vi "TDT-Stream AO.vi"(0 "RPcox":refnum<k7>, 2 "Action":T1=enum."Write", 5 "Restart":bool, 7 "Output array":dbl[][](array[numeric]), 9 "Chans":i32[](array[numeric]), 11 "error in (no error)":errorcluster) -> (4 "RPcox thru":refnum<k7>, 15 "error out":errorcluster={"status"=FALSE, "code"=0, "source"="."})   [LabVIEW 2020]
uses:
  TDT-Signal Bank Action.ctl
  TDT-Globals.vi
  Utility VIs/Array Manipulation VIs/Array-Dimensions (2D).vi
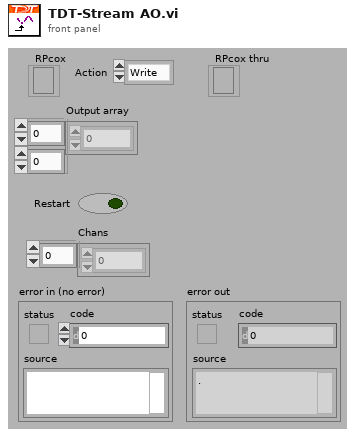
[diagram p1: front panel]
types:
  T1 = typedef "TDT-Signal Bank Action.ctl" = enum16{"Init", "Write", "Read", "Rewrite", "Reset", "Recycle", "Ramp up", "Ramp down", "Zero"}
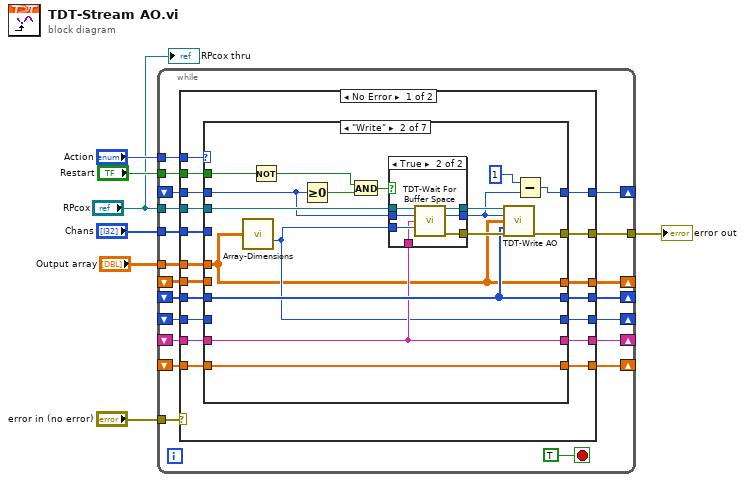
[diagram p0: block diagram]
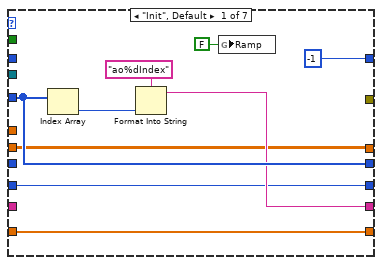
[diagram p2: hidden frame]
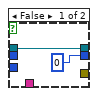
[diagram p3: hidden frame]
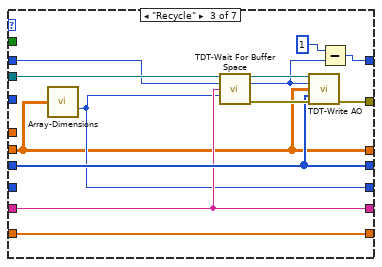
[diagram p4: hidden frame]
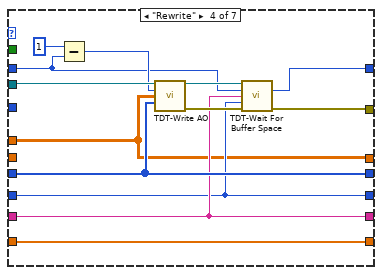
[diagram p5: hidden frame]
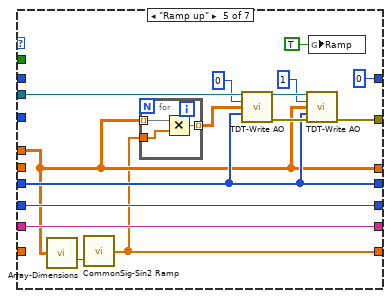
[diagram p6: hidden frame]
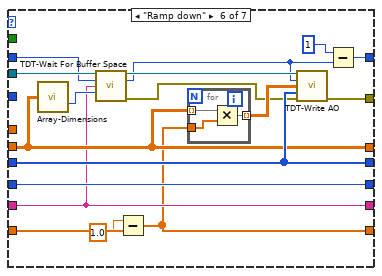
[diagram p7: hidden frame]
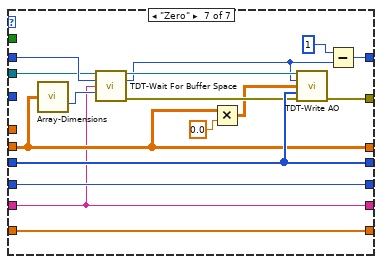
[diagram p8: hidden frame]
diagram:
  n1 = while {
    tunnel: [w27] -> w7
    tunnel: "error in (no error)" -> [w26]
    tunnel: "RPcox" -> [w25]
    tunnel: "Action" -> [w23]
    shift-right: [w21] -> _
    shift-left: _ -> [w20]
    tunnel: "Chans" -> [w19]
    shift-right: [w18] -> _
    shift-left: _ -> [w17]
    shift-right: [w16] -> _
    shift-left: _ -> [w15]
    shift-right: [w14] -> _
    shift-left: _ -> [w13]
    shift-right: [w12] -> _
    shift-left: _ -> [w24]
    shift-right: [w11] -> _
    shift-left: _ -> [w10]
    tunnel: "Output array" -> [w9]
    tunnel: "Restart" -> [w8]
    stop <- TRUE stop-if-true
    n2 = case shown="No Error" w26 {
      selector: w26 -> [_ w167]
      tunnel: [w40 w167] -> w27
      tunnel: w25 -> [w41 _]
      tunnel: w24 -> [w45 w162]
      tunnel: w23 -> [w44 _]
      tunnel: [w43 w166] -> w21
      tunnel: w20 -> [w42 w166]
      tunnel: w19 -> [w39 _]
      tunnel: [w38 w165] -> w18
      tunnel: w17 -> [w37 w165]
      tunnel: [w36 w164] -> w16
      tunnel: w15 -> [w35 w164]
      tunnel: [w34 w163] -> w14
      tunnel: w13 -> [w33 w163]
      tunnel: [w32 w162] -> w12
      tunnel: [w31 w161] -> w11
      tunnel: w10 -> [w30 w161]
      tunnel: w9 -> [w29 _]
      tunnel: w8 -> [w28 _]
      frame No Error {
        n3 = case shown="\"Write\"" w44 {
          tunnel: w45 -> [w48 _ w81 _ _ w137 w157]
          tunnel: [-1 w71 w93 w105 0 ("Next Buffer Out") w129 w149] -> w43
          tunnel: w42 -> [_ w64 w86 w99 _ w138 w158]
          tunnel: w41 -> [_ w68 w90 w103 w118 w139 w145]
          tunnel: [_ w66 w88 w96 w114 w125 w154] -> w40
          tunnel: w39 -> [w52 _ _ _ _ _ _]
          tunnel: [w52 w62 w85 w101 w111 w140 w159] -> w38
          tunnel: w37 -> [_ w62 w85 w101 w111 w140 w159]
          tunnel: [w50 w61 w84 w98 w120 w135 w155] -> w36
          tunnel: w35 -> [_ w61 w84 w98 w120 w135 w155]
          tunnel: [w49 w60 w83 w97 w121 w141 w160] -> w34
          tunnel: w33 -> [w49 _ _ w97 w121 w141 w160]
          tunnel: [w48 w58 w81 w94 w109 w137 w157] -> w32
          tunnel: [w47 w59 w82 w95 w107 w133 w153] -> w31
          tunnel: w30 -> [w47 w59 w82 w95 _ w134 w153]
          tunnel: w29 -> [_ w58 _ w94 w109 _ _]
          tunnel: w28 -> [_ w56 _ _ _ _ _]
          frame "Init", Default {
            n4 = Index Array(array=w52) -> (element=w51:i32)  [unwired: 1 in]
            n5 = Format Into String(format string="ao%dIndex", w51) -> (resulting string=w50:string)  [unwired: 2 in, 1 out]
            n6 = global write "TDT-Globals.vi" "Ramp"(FALSE ("Ramp")) -> ()
          }
          frame "Write" {
            n7 = call-poly "Array-Dimensions.vi"("2D Array"=w58) -> ("# columns"=w60:i32)  [unwired: 13 in, 1 out]
            n8 = Not(x=w56) -> (.not. x?=w55:bool)
            n9 = Greater Or Equal To 0?(x=w64) -> (x >= 0?=w63:bool)
            n10 = And(x=w55, y=w63) -> (x .and. y?=w57:bool)
            n11 = case shown="True" w57 {
              tunnel: [_ w80] -> w69
              tunnel: w68 -> [w73 w79]
              tunnel: [w73 w78] -> w67
              tunnel: w64 -> [_ w77]
              tunnel: w60 -> [_ w76]
              tunnel: [0 ("Next Buffer Out") w75] -> w65
              tunnel: w61 -> [_ w74]
              frame False {
              }
              frame True {
                n12 = call "TDT-Wait For Buffer Space.vi"("RPcox"=w79, "Next Buffer"=w77, "Tag"=w74, "Buffer Length"=w76) -> ("RPcox Out"=w78:refnum<k7>, "Next Buffer thru"=w75:i32, "error out"=w80:errorcluster)  [unwired: 9 in]
              }
            }
            n13 = call "TDT-Write AO.vi"("RPcox"=w67, "Next Buffer"=w65, "Input array"=w58, "Chans"=w62, "error in (no error)"=w69) -> ("error out"=w66:errorcluster)  [unwired: 9 in, 1 out]
            n14 = Subtract(x=1, y=w65) -> (x-y=w71:i32)
          }
          frame "Recycle" {
            n15 = call-poly "Array-Dimensions.vi"("2D Array"=w81) -> ("# columns"=w83:i32)  [unwired: 13 in, 1 out]
            n16 = call "TDT-Wait For Buffer Space.vi"("RPcox"=w90, "Next Buffer"=w86, "Tag"=w84, "Buffer Length"=w83) -> ("RPcox Out"=w89:refnum<k7>, "Next Buffer thru"=w87:i32, "error out"=w91:errorcluster)  [unwired: 9 in]
            n17 = call "TDT-Write AO.vi"("RPcox"=w89, "Next Buffer"=w87, "Input array"=w81, "Chans"=w85, "error in (no error)"=w91) -> ("error out"=w88:errorcluster)  [unwired: 9 in, 1 out]
            n18 = Subtract(x=1, y=w87) -> (x-y=w93:i32)
          }
          frame "Rewrite" {
            n19 = Subtract(x=1, y=w99) -> (x-y=w102:i32)
            n20 = call "TDT-Write AO.vi"("RPcox"=w103, "Next Buffer"=w102, "Input array"=w94, "Chans"=w101) -> ("RPcox (thru)"=w100:refnum<k7>, "error out"=w104:errorcluster)  [unwired: 10 in]
            n21 = call "TDT-Wait For Buffer Space.vi"("RPcox"=w100, "Next Buffer"=w99, "Tag"=w98, "Buffer Length"=w97, "error in (no error)"=w104) -> ("Next Buffer thru"=w105:i32, "error out"=w96:errorcluster)  [unwired: 8 in, 1 out]
          }
          frame "Ramp up" {
            n22 = call-poly "Array-Dimensions.vi"("2D Array"=w109) -> ("# columns"=w108:i32)  [unwired: 13 in, 1 out]
            n23 = call "CommonSig-Sin2 Ramp.vi"("samples"=w108) -> ("sine^2 Ramp"=w107:dbl[])  [unwired: 3 in, 1 out]
            n24 = for {
              tunnel: w109 -> [w124] mode=indexing
              tunnel: [w123] -> w110 mode=indexing
              tunnel: w107 -> [w122]
              n25 = Multiply(x=w124, y=w122) -> (x*y=w123:dbl[])
            }
            n26 = call "TDT-Write AO.vi"("RPcox"=w118, "Next Buffer"=0, "Input array"=w110, "Chans"=w111) -> ("RPcox (thru)"=w113:refnum<k7>, "error out"=w115:errorcluster)  [unwired: 10 in]
            n27 = call "TDT-Write AO.vi"("RPcox"=w113, "Next Buffer"=1, "Input array"=w109, "Chans"=w111, "error in (no error)"=w115) -> ("error out"=w114:errorcluster)  [unwired: 9 in, 1 out]
            n28 = global write "TDT-Globals.vi" "Ramp"(TRUE ("Ramp")) -> ()
          }
          frame "Ramp down" {
            n29 = call-poly "Array-Dimensions.vi"("2D Array"=w137) -> ("# columns"=w136:i32)  [unwired: 13 in, 1 out]
            n30 = call "TDT-Wait For Buffer Space.vi"("RPcox"=w139, "Next Buffer"=w138, "Tag"=w135, "Buffer Length"=w136) -> ("RPcox Out"=w131:refnum<k7>, "Next Buffer thru"=w128:i32, "error out"=w126:errorcluster)  [unwired: 9 in]
            n31 = Subtract(x=1.0, y=w134) -> (x-y=w133:dbl[])
            n32 = for {
              tunnel: w137 -> [w144] mode=indexing
              tunnel: [w143] -> w127 mode=indexing
              tunnel: w133 -> [w142]
              n33 = Multiply(x=w144, y=w142) -> (x*y=w143:dbl[])
            }
            n34 = call "TDT-Write AO.vi"("RPcox"=w131, "Next Buffer"=w128, "Input array"=w127, "Chans"=w140, "error in (no error)"=w126) -> ("error out"=w125:errorcluster)  [unwired: 9 in, 1 out]
            n35 = Subtract(x=1, y=w128) -> (x-y=w129:i32)
          }
          frame "Zero" {
            n36 = call-poly "Array-Dimensions.vi"("2D Array"=w157) -> ("# columns"=w156:i32)  [unwired: 13 in, 1 out]
            n37 = call "TDT-Wait For Buffer Space.vi"("RPcox"=w145, "Next Buffer"=w158, "Tag"=w155, "Buffer Length"=w156) -> ("RPcox Out"=w152:refnum<k7>, "Next Buffer thru"=w147:i32, "error out"=w151:errorcluster)  [unwired: 9 in]
            n38 = Multiply(x=w157, y=0.0) -> (x*y=w146:dbl[][])
            n39 = call "TDT-Write AO.vi"("RPcox"=w152, "Next Buffer"=w147, "Input array"=w146, "Chans"=w159, "error in (no error)"=w151) -> ("error out"=w154:errorcluster)  [unwired: 9 in, 1 out]
            n40 = Subtract(x=1, y=w147) -> (x-y=w149:i32)
          }
        }
      }
      frame Error {
      }
    }
  }
  "error out" <- w7
  "RPcox thru" <- "RPcox"
